vi "Parse Sensor Group 3.vi"(11 "stream in":u8[](array[numeric])) -> (1 "Sensor Group 3":T1, 3 "stream out":u8[](array[numeric]))   [LabVIEW 2013]
doc: "Read Sensor Group 3 from a UART data stream."
uses:
  Sensor Group 3.ctl
  Charging State.ctl
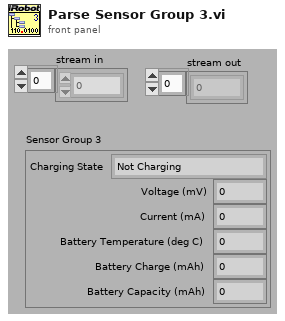
[diagram p1: front panel]
types:
  T1 = typedef "Sensor Group 3.ctl" = cluster{"Charging State":T2, "Voltage (mV)":u16, "Current (mA)":i16, "Battery Temperature (deg C)":i8, "Battery Charge (mAh)":u16, "Battery Capacity (mAh)":u16}
  T2 = typedef "Charging State.ctl" = enum16{"Not Charging", "Reconditioning Charging", "Full Charging", "Trickle Charging", "Waiting", "Charging Fault Condition"}
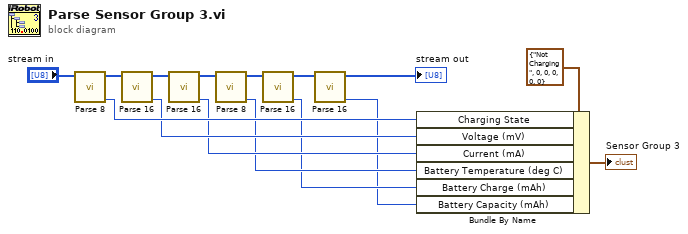
[diagram p0: block diagram]
diagram:
  n1 = call "Parse 8.vi"("stream in"="stream in") -> ("value"=w12:u8, "stream out"=w11:u8[])  [unwired: 9 out]
  n2 = call "Parse 16.vi"("stream in"=w11) -> ("value"=w10:u16, "stream out"=w9:u8[])  [unwired: 9 out]
  n3 = call "Parse 16.vi"("stream in"=w9) -> ("value"=w8:u16, "stream out"=w7:u8[])  [unwired: 9 out]
  n4 = call "Parse 8.vi"("stream in"=w7) -> ("value"=w6:u8, "stream out"=w5:u8[])  [unwired: 9 out]
  n5 = call "Parse 16.vi"("stream in"=w5) -> ("value"=w4:u16, "stream out"=w3:u8[])  [unwired: 9 out]
  n6 = call "Parse 16.vi"("stream in"=w3) -> ("value"=w2:u16, "stream out"=→"stream out":u8[])  [unwired: 9 out]
  n7 = Bundle By Name(cluster=T1 {"Charging State"=enum."Not Charging", "Voltage (mV)"=0, "Current (mA)"=0, "Battery Temperature (deg C)"=0, "Battery Charge (mAh)"=0, "Battery Capacity (mAh)"=0} ("Sensor Group 3"), "Charging State"=w12, "Voltage (mV)"=w10, "Current (mA)"=w8, "Battery Temperature (deg C)"=w6, "Battery Charge (mAh)"=w4, "Battery Capacity (mAh)"=w2) -> (→"Sensor Group 3":T1)
